vi "BK Precision 9200 Voltage Control Test.vi"() -> ()   [LabVIEW 2017]
doc: "This example shows how to configure the instrument's output voltage level and over voltage protection. The actual voltage level and actual current level are returned."
uses:
  Downloads/bk_precision_9200_series/BK Precision 9200 Series/BK Precision 9200 Series.lvlib
panel:
  in  "Boolean":bool
  in  "Sampling Interval (s)":i32=30
  in  "Duration Off (m)":i32=30
  in  "Duration On (m)":i32=90
  out "Current Current (mA)":dbl
  out "Current Voltage (V)":dbl
  in  "Current Limit (1.0 A)":dbl=1.0 format="%.3g"
  in  "Enable OVP (T: Enable)":bool=TRUE
  in  "Stop Output":bool
  in  "Voltage Limit (66V)":dbl=66.0 format="%.2f"
  in  "Voltage Level (1.0 V)":dbl=1.0 format="%.3f"
  in  "VISA resource name":refnum<visa-resource-name>
  # "(c) 2014 B&K Precision Corporation.  ALL RIGHTS RESERVED."
  # "Over Voltage Protection"
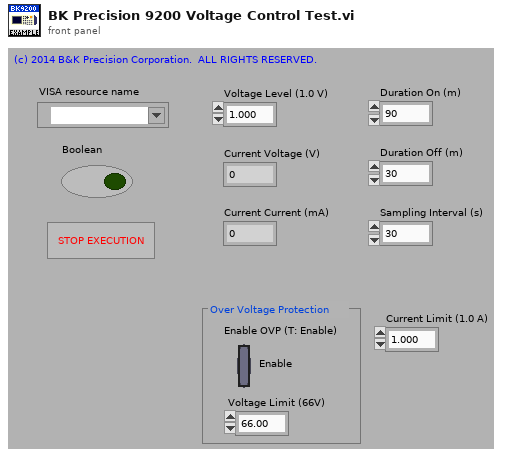
[diagram p1: front panel]
types:
  T1 = enum16{"open", "replace", "create", "open or create", "replace or create", "replace or create with confirmation"}
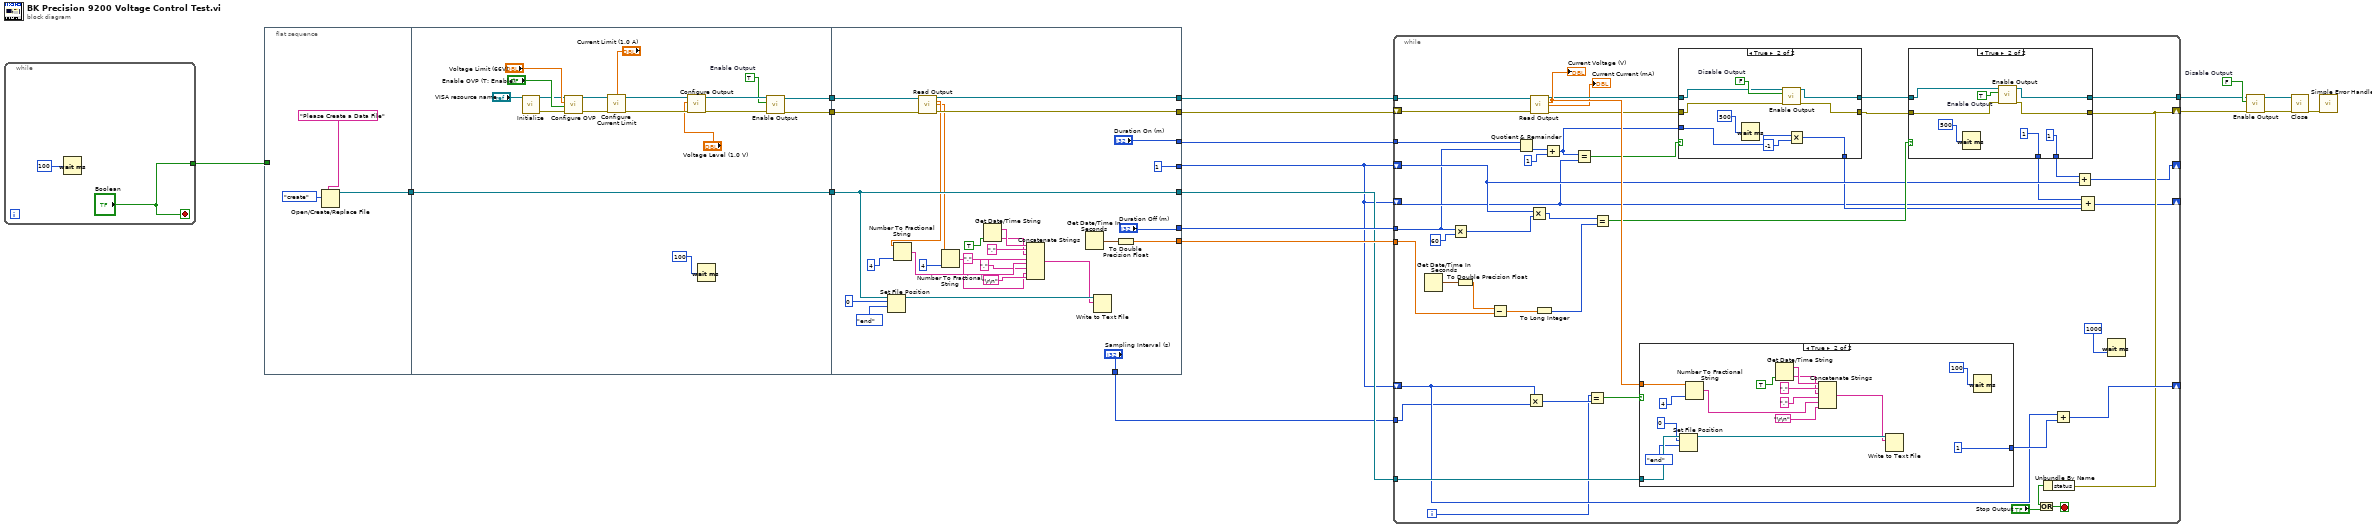
[diagram p0: block diagram]
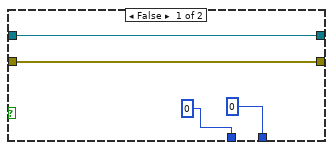
[diagram p2: hidden frame]
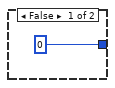
[diagram p3: hidden frame]
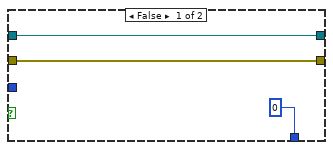
[diagram p4: hidden frame]
diagram:
  w5 = FALSE  # Disable Output
  n1 = while {
    tunnel: ["Boolean"] -> w6
    stop <- "Boolean" stop-if-true
    n2 = Wait (ms)(milliseconds to wait=100) -> ()  [unwired: 1 out]
  }
  n3 = flat-sequence {
    tunnel: [w23] -> w11
    tunnel: w6 -> [_]
    tunnel: [w28] -> w13
    tunnel: [w27] -> w12
    tunnel: w11 -> [w26]
    tunnel: [w26] -> w10
    tunnel: ["Duration Off (m)"] -> w14
    tunnel: ["Duration On (m)"] -> w15
    tunnel: [w65] -> w16
    tunnel: [1] -> w7
    tunnel: [w67] -> w17
    tunnel: [w68] -> w18
    tunnel: w13 -> [w70]
    tunnel: w12 -> [w69]
    tunnel: w10 -> [w50]
    tunnel: [w50] -> w9
    tunnel: ["Sampling Interval (s)"] -> w8
    frame #0 {
      n4 = Open/Create/Replace File(prompt="Please Create a Data File", operation (0:open)=T1."create") -> (refnum out=w23:refnum<file>)  [unwired: 4 in, 2 out]
    }
    frame #1 {
      w29 = TRUE  # Enable Output
      n5 = call "Initialize.vi"("VISA resource name"="VISA resource name") -> ("error out"=w31:errorcluster, "VISA resource name out"=w32:refnum<visa-resource-name>)  [unwired: 9 in]
      n6 = call "Configure OVP.vi"("error in (no error)"=w31, "Enable OVP (T: Enable)"="Enable OVP (T: Enable)", "Voltage Limit (66.000 V)"="Voltage Limit (66V)", "VISA resource name"=w32) -> ("error out"=w37:errorcluster, "VISA resource name out"=w36:refnum<visa-resource-name>)  [unwired: 6 in]
      n7 = call "Configure Current Limit.vi"("error in (no error)"=w37, "Current Limit (0.0 A)"="Current Limit (1.0 A)", "VISA resource name"=w36) -> ("error out"=w40:errorcluster, "VISA resource name out"=w39:refnum<visa-resource-name>)  [unwired: 7 in]
      n8 = call "Configure Output.vi"("error in (no error)"=w40, "Voltage Level (0.0 V)"="Voltage Level (1.0 V)", "VISA resource name"=w39) -> ("error out"=w42:errorcluster, "VISA resource name out"=w41:refnum<visa-resource-name>)  [unwired: 7 in]
      n9 = Wait (ms)(milliseconds to wait=100) -> ()  [unwired: 1 out]
      n10 = call "Enable Output.vi"("error in (no error)"=w42, "Enable Output (F: False)"=w29, "VISA resource name"=w41) -> ("error out"=w27:errorcluster, "VISA resource name out"=w28:refnum<visa-resource-name>)  [unwired: 7 in]
    }
    frame #2 {
      n11 = Set File Position(offset (in bytes) (0)=i64 0, refnum=w50, from (0:start)=enum16{"start", "end", "current"}."end") -> (refnum out=w59:refnum<file>)  [unwired: 1 in, 1 out]
      n12 = call "Read Output.vi"("VISA resource name"=w70, "error in (no error)"=w69) -> ("VISA resource name out"=w68:refnum<visa-resource-name>, "Actual Voltage Level (V)"=w48:dbl, "Actual Current Level (A)"=w47:dbl, "error out"=w67:errorcluster)  [unwired: 9 in, 1 out]
      n13 = Number To Fractional String(number=w48, precision (6)=4) -> (F-format string=w53:string)  [unwired: 2 in]
      n14 = Number To Fractional String(number=w47, precision (6)=4) -> (F-format string=w43:string)  [unwired: 2 in]
      n15 = Get Date/Time String(want seconds? (F)=TRUE) -> (date string=w57:string, time string=w55:string)  [unwired: 2 in]
      n16 = Concatenate Strings(w57, ",", w55, ",", w53, ",", w43, "\r\n") -> (w58:string)
      n17 = Get Date/Time In Seconds() -> (seconds since 1Jan1904=w66:timestamp)
      n18 = Write to Text File(file (use dialog)=w59, text=w58) -> ()  [unwired: 2 in, 3 out]
      n19 = To Double Precision Float(number=w66) -> (double precision float=w65:dbl)
    }
  }
  n20 = while {
    shift-right: [w93] -> w3
    shift-left: w17 -> [w91]
    tunnel: [w94] -> w4
    tunnel: w16 -> [w109]
    shift-right: [w86] -> _
    shift-left: w7 -> [w87]
    tunnel: w9 -> [w103]
    shift-right: [w101] -> _
    shift-left: w7 -> [w99]
    tunnel: w18 -> [w92]
    shift-right: [w84] -> _
    shift-left: w7 -> [w82]
    tunnel: w14 -> [w73]
    tunnel: w15 -> [w74]
    tunnel: w8 -> [w72]
    i -> [w71]
    stop <- w114 stop-if-true
    n21 = Get Date/Time In Seconds() -> (seconds since 1Jan1904=w110:timestamp)
    n22 = Multiply(x=w73, y=60) -> (x*y=w78:i32)
    n23 = To Double Precision Float(number=w110) -> (double precision float=w108:dbl)
    n24 = Subtract(x=w108, y=w109) -> (x-y=w107:dbl)
    n25 = Quotient & Remainder(x=w74, y=w73) -> (floor(x/y)=w77:i32)  [unwired: 1 out]
    n26 = Multiply(x=w99, y=w72) -> (x*y=w105:i32)
    n27 = call "Read Output.vi"("VISA resource name"=w92, "error in (no error)"=w91) -> ("VISA resource name out"=w98:refnum<visa-resource-name>, "Actual Voltage Level (V)"=w102:dbl, "Actual Current Level (A)"=→"Current Current (mA)":dbl, "error out"=w97:errorcluster)  [unwired: 9 in, 1 out]
    "Current Voltage (V)" <- w102
    n28 = Multiply(x=w87, y=w78) -> (x*y=w106:i32)
    n29 = To Long Integer(number=w107) -> (32bit integer=w90:i32)
    n30 = Add(x=w77, y=1) -> (x+y=w75:i32)
    n31 = Equal?(x=w75, y=w82) -> (x = y?=w81:bool)
    n32 = Equal?(x=w71, y=w105) -> (x = y?=w104:bool)
    n33 = Equal?(x=w106, y=w90) -> (x = y?=w89:bool)
    n34 = case shown="True" w104 {
      tunnel: w103 -> [_ w140]
      tunnel: w102 -> [_ w143]
      tunnel: [0 1] -> w100
      frame False {
      }
      frame True {
        n35 = Set File Position(offset (in bytes) (0)=i64 0, refnum=w140, from (0:start)=enum16{"start", "end", "current"}."end") -> (refnum out=w137:refnum<file>)  [unwired: 1 in, 1 out]
        n36 = Number To Fractional String(number=w143, precision (6)=4) -> (F-format string=w131:string)  [unwired: 2 in]
        n37 = Get Date/Time String(want seconds? (F)=TRUE) -> (date string=w135:string, time string=w133:string)  [unwired: 2 in]
        n38 = Concatenate Strings(w135, ",", w133, ",", w131, "\r\n") -> (w136:string)
        n39 = Write to Text File(file (use dialog)=w137, text=w136) -> ()  [unwired: 2 in, 3 out]
        n40 = Wait (ms)(milliseconds to wait=100) -> ()  [unwired: 1 out]
      }
    }
    n41 = case shown="True" w81 {
      tunnel: w98 -> [w146 w153]
      tunnel: w97 -> [w145 w152]
      tunnel: [w146 w151] -> w95
      tunnel: [w145 w150] -> w96
      tunnel: [0 w148] -> w83
      tunnel: w75 -> [_ w149]
      frame False {
      }
      frame True {
        w154 = FALSE  # Disable Output
        n42 = Wait (ms)(milliseconds to wait=500) -> ()  [unwired: 1 out]
        n43 = call "Enable Output.vi"("error in (no error)"=w152, "Enable Output (F: False)"=w154, "VISA resource name"=w153) -> ("error out"=w150:errorcluster, "VISA resource name out"=w151:refnum<visa-resource-name>)  [unwired: 7 in]
        n44 = Multiply(x=w149, y=-1) -> (x*y=w148:i32)
      }
    }
    n45 = case shown="True" w89 {
      tunnel: w96 -> [w118 w123]
      tunnel: [w118 w121] -> w93
      tunnel: w95 -> [w117 w124]
      tunnel: [w117 w122] -> w94
      tunnel: [0 1] -> w88
      tunnel: [0 1] -> w85
      frame False {
      }
      frame True {
        w125 = TRUE  # Enable Output
        n46 = Wait (ms)(milliseconds to wait=500) -> ()  [unwired: 1 out]
        n47 = call "Enable Output.vi"("error in (no error)"=w123, "Enable Output (F: False)"=w125, "VISA resource name"=w124) -> ("error out"=w121:errorcluster, "VISA resource name out"=w122:refnum<visa-resource-name>)  [unwired: 7 in]
      }
    }
    n48 = Unbundle By Name(w93) -> ("status"=w112:bool)
    n49 = Or(x=w112, y="Stop Output") -> (x .or. y?=w114:bool)
    n50 = Add(x=w99, y=w100) -> (x+y=w101:i32)
    n51 = Add(x=w88, y=w87) -> (x+y=w86:i32)
    n52 = Compound Arithmetic op=ADD(w85, w82, w83) -> (w84:i32)
    n53 = Wait (ms)(milliseconds to wait=1000) -> ()  [unwired: 1 out]
  }
  n54 = call "Enable Output.vi"("error in (no error)"=w3, "Enable Output (F: False)"=w5, "VISA resource name"=w4) -> ("error out"=w1:errorcluster, "VISA resource name out"=w2:refnum<visa-resource-name>)  [unwired: 7 in]
  n55 = call "Close.vi"("error in (no error)"=w1, "VISA resource name"=w2) -> ("error out"=w19:errorcluster)  [unwired: 9 in]
  n56 = call <vilib>:"Simple Error Handler.vi"("error in (no error)"=w19) -> ()  [unwired: 4 in, 5 out]
